vi "calcForceMeasured.vi"(8 "error in (no error)":errorcluster, 11 "ForceSensor in":refnum<class "ForceSensorCalculator.lvclass">) -> (0 "error out":errorcluster, 3 "ForceSensor out":refnum<class "ForceSensorCalculator.lvclass">)   [LabVIEW 2013, in "ForceSensorCalculator.lvlib" / "ForceSensorCalculator.lvclass"]
uses:
  <userlib>/Common/Devices/ForceSensorCalculator/ForceSensorCalculator/ForceSensorCalculator.lvclass
  <userlib>/Common/Devices/ForceSensorCalculator/ForceSensorCalculator/ForceSensorCalculator.lvclass/ForceSensorCalculator.ctl
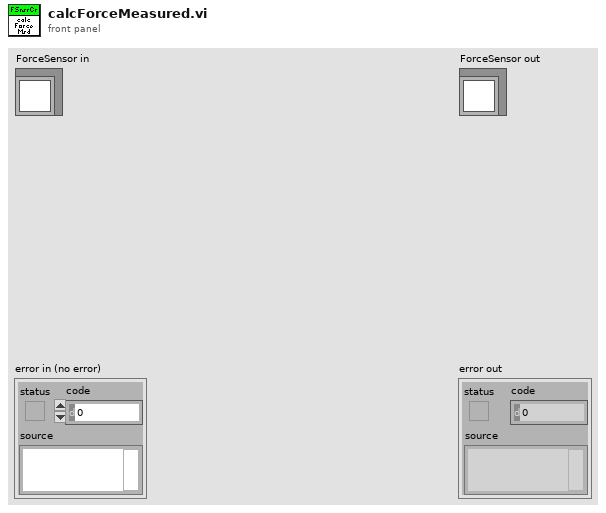
[diagram p1: front panel]
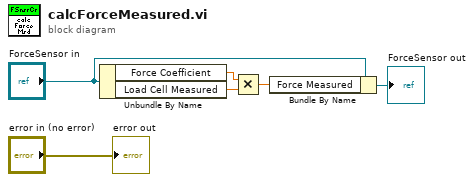
[diagram p0: block diagram]
diagram:
  n1 = Unbundle By Name("ForceSensor in") -> ("Force Coefficient"=w3:dbl[unit], "Load Cell Measured"=w2:dbl[unit])
  n2 = Multiply(x=w3, y=w2) -> (x*y=w1:dbl[unit])
  n3 = Bundle By Name(cluster="ForceSensor in", "Force Measured"=w1) -> (→"ForceSensor out":refnum<class "ForceSensorCalculator.lvclass">)
  "error out" <- "error in (no error)"
